vi "AutoConvertString2Numeric.vi"(8 "error in (no error)":errorcluster, 11 "string in":string) -> (0 "error out":errorcluster, 3 "Numeric out":dbl format="%#_26g")   [LabVIEW 2016, in "Dxf.lvlib"]
uses:
  Dxf.lvlib
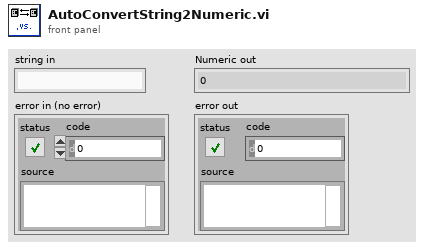
[diagram p1: front panel]
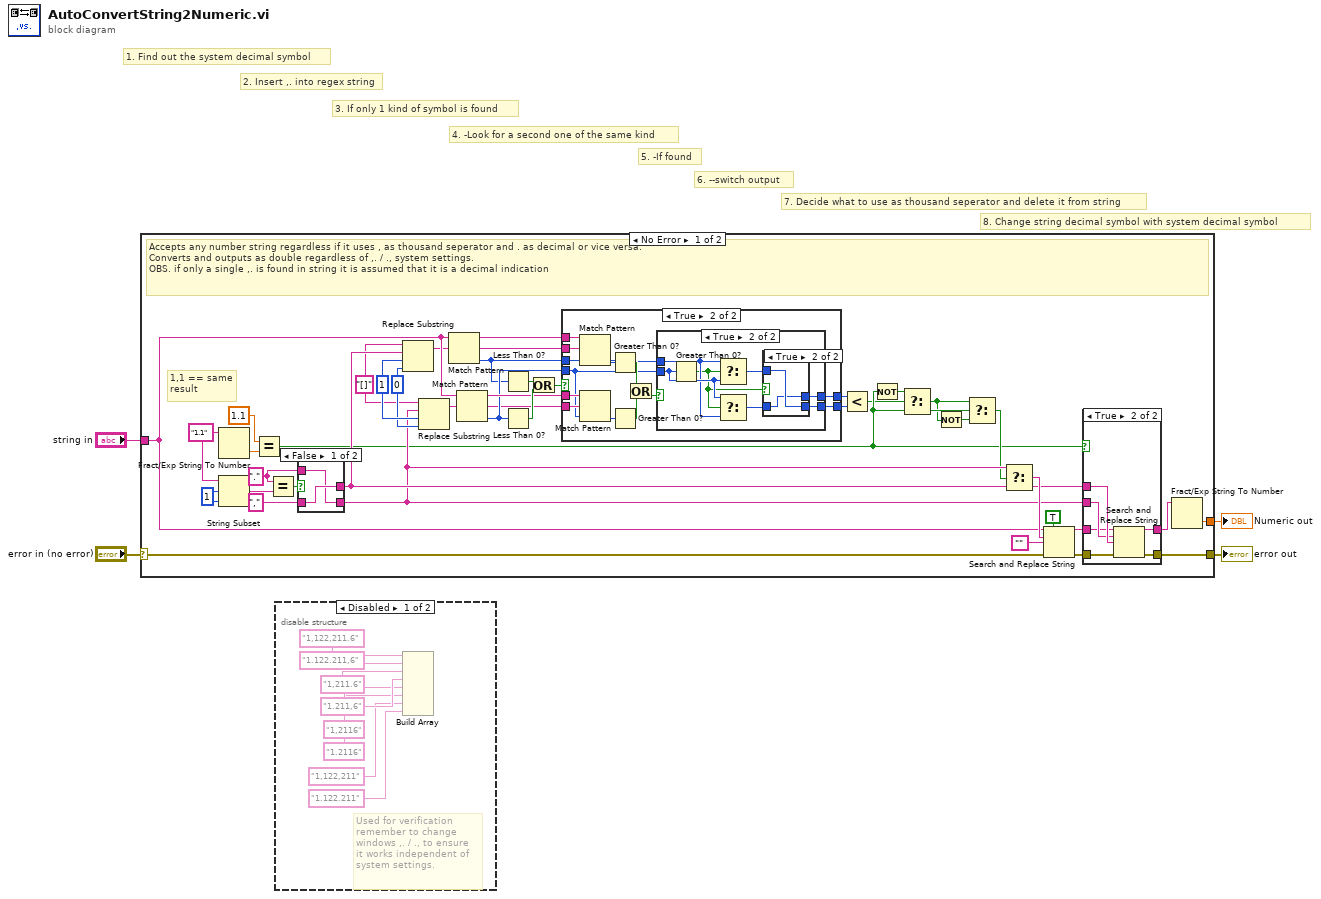
[diagram p0: block diagram]
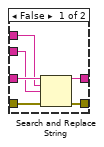
[diagram p7: hidden frame]
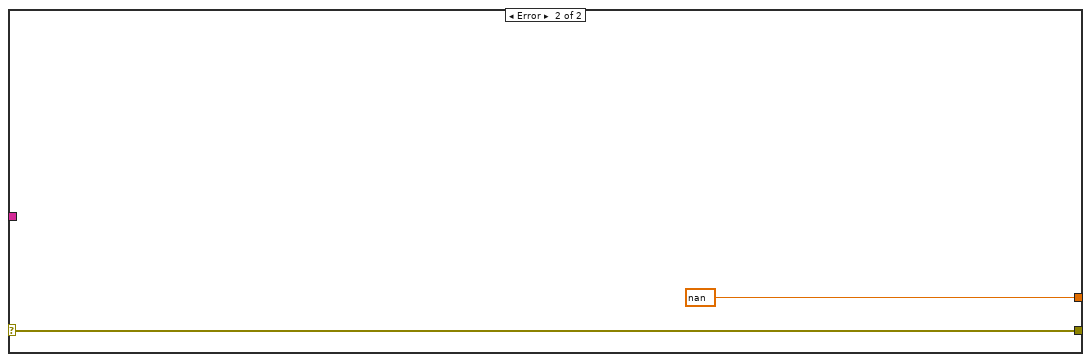
[diagram p8: hidden frame]
diagram:
  # "8. Change string decimal symbol with system decimal symbol"
  # "6. --switch output"
  # "5. -If found"
  # "4. -Look for a second one of the same kind"
  # "3. If only 1 kind of symbol is found"
  # "2. Insert ,. into regex string"
  # "1. Find out the system decimal symbol"
  # "7. Decide what to use as thousand seperator and delete it from string"
  n1 = case shown="No Error" "error in (no error)" {
    selector: "error in (no error)" -> [w20 w88]
    tunnel: "string in" -> [w15 _]
    tunnel: [w22 nan] -> w3
    tunnel: [w19 w88] -> w1
    frame No Error {
      w29 = 0 ("length (len. of substring)")
      w30 = 1 ("offset (0)")
      w21 = "[]" ("regular expression")
      w27 = "." ("string")
      w35 = 1 ("offset (0)")
      w34 = "1.1" ("string")
      # "1,1 == same\nresult"
      # "Accepts any number string regardless if it uses , as thousand seperator and . as decimal or vice versa.\nConverts and outputs as double regardless of ,. / ., system settings.\nOBS. if only a single ,. is found in string it is assumed that it is a decimal indication"
      n2 = Fract/Exp String To Number(string=w34) -> (number=w31:dbl)  [unwired: 3 in, 1 out]
      n3 = String Subset(string=w34, offset (0)=w35, length (rest)=w35) -> (substring=w36:string)
      n4 = Equal?(x=1.1 ("number"), y=w31) -> (x = y?=w23:bool)
      n5 = Equal?(x=w27, y=w36) -> (x = y?=w42:bool)
      n6 = case shown="False" w42 {
        tunnel: [w72 w74] -> w26
        tunnel: w27 -> [w71 w74]
        tunnel: [w71 w73] -> w25
        tunnel: "," ("string") -> [w72 w73]
        frame False {
        }
        frame True {
        }
      }
      n7 = Replace Substring(2:w29, 3:w30, 4:w26, 5:w21) -> (1:w6:string)  [unwired: 1 out]
      n8 = Replace Substring(2:w29, 3:w30, 4:w25, 5:w21) -> (1:w5:string)  [unwired: 1 out]
      n9 = Match Pattern(string=w15, regular expression=w6) -> (offset past match=w13:i32)  [unwired: 1 in, 3 out]
      n10 = Match Pattern(string=w15, regular expression=w5) -> (offset past match=w14:i32)  [unwired: 1 in, 3 out]
      n11 = Less Than 0?(x=w13) -> (x < 0?=w18:bool)
      n12 = Less Than 0?(x=w14) -> (x < 0?=w17:bool)
      n13 = Or(x=w18, y=w17) -> (x .or. y?=w16:bool)
      n14 = case shown="True" w16 {
        tunnel: w15 -> [_ w57]
        tunnel: w15 -> [_ w56]
        tunnel: w14 -> [w43 w45]
        tunnel: w13 -> [w44 w47]
        tunnel: [w44 w48] -> w12
        tunnel: [w43 w46] -> w11
        tunnel: w6 -> [_ w55]
        tunnel: w5 -> [_ w54]
        frame False {
        }
        frame True {
          n15 = Match Pattern(string=w57, regular expression=w55, offset (0)=w47) -> (offset past match=w53:i32)  [unwired: 3 out]
          n16 = Match Pattern(string=w56, regular expression=w54, offset (0)=w45) -> (offset past match=w52:i32)  [unwired: 3 out]
          n17 = Greater Than 0?(x=w53) -> (x > 0?=w50:bool)
          n18 = Greater Than 0?(x=w52) -> (x > 0?=w49:bool)
          n19 = Or(x=w50, y=w49) -> (x .or. y?=w51:bool)
          n20 = case shown="True" w51 {
            tunnel: [w59 w63] -> w48
            tunnel: w47 -> [w59 w65]
            tunnel: [w58 w61] -> w46
            tunnel: w45 -> [w58 w66]
            frame False {
            }
            frame True {
              n21 = Greater Than 0?(x=w66) -> (x > 0?=w64:bool)
              n22 = Select(t=w65, s=w64, f=w66) -> (s? t:f=w62:i32)
              n23 = Select(t=w66, s=w64, f=w65) -> (s? t:f=w60:i32)
              n24 = case shown="True" w64 {
                tunnel: [w68 w69] -> w63
                tunnel: w62 -> [w68 w70]
                tunnel: [w67 w70] -> w61
                tunnel: w60 -> [w67 w69]
                frame False {
                }
                frame True {
                }
              }
            }
          }
        }
      }
      n25 = Less?(x=w12, y=w11) -> (x < y?=w10:bool)
      n26 = Not(x=w23) -> (.not. x?=w9:bool)
      n27 = Select(t=w9, s=w10, f=w23) -> (s? t:f=w8:bool)
      n28 = Not(x=w8) -> (.not. x?=w7:bool)
      n29 = Select(t=w8, s=w23, f=w7) -> (s? t:f=w24:bool)
      n30 = Select(t=w25, s=w24, f=w26) -> (s? t:f=w41:string)
      n31 = Search and Replace String(replace all?=TRUE ("replace all? (F)"), input string=w15, search string=w41, replace string="", error in=w20) -> (result string=w38:string, error out=w39:errorcluster)  [unwired: 3 in, 2 out]
      n32 = case shown="True" w23 {
        tunnel: [w80 w85] -> w19
        tunnel: w38 -> [w79 w82]
        tunnel: w39 -> [w78 w86]
        tunnel: w26 -> [w77 w84]
        tunnel: w25 -> [w76 w83]
        tunnel: [w75 w81] -> w33
        frame False {
          n33 = Search and Replace String(input string=w79, search string=w77, replace string=w76, error in=w78) -> (result string=w75:string, error out=w80:errorcluster)  [unwired: 4 in, 2 out]
        }
        frame True {
          n34 = Search and Replace String(input string=w82, search string=w83, replace string=w84, error in=w86) -> (result string=w81:string, error out=w85:errorcluster)  [unwired: 4 in, 2 out]
        }
      }
      n35 = Fract/Exp String To Number(string=w33) -> (number=w22:dbl)  [unwired: 3 in, 1 out]
    }
    frame Error {
    }
  }
  "Numeric out" <- w3
  "error out" <- w1
  n36 = disable-structure shown="Disabled" {
    frame Disabled {
      # "Used for verification\nremember to change\nwindows ,. / ., to ensure\nit works independent of\nsystem settings."
      n37 = Build Array("1,122,211.6" ("string in 2"), "1.122.211,6" ("string in 2"), "1,211.6" ("string in 2"), "1.211,6" ("string in 2"), "1,2116" ("string in 2"), "1.2116" ("string in 2"), "1,122,211" ("string in 2"), "1.122.211" ("string in 2")) -> ()  [unwired: 1 out]
    }
    frame Enabled {
    }
  }
